vi "Kepco cfg run list.vi"(8 "error in (no error)":errorcluster {"code" format="%.0x"}, 9 "Simulation":T1, 10 "Channel parsed command info":T2, 11 "input cluster":refnum<class "KepcoBOP.lvclass">) -> (0 "error out":errorcluster, 2 "new commands":string, 3 "output cluster":refnum<class "KepcoBOP.lvclass">)   [LabVIEW 2020, in "KepcoBOP.lvclass"]
uses:
  KepcoBOP.lvclass
  channel parsed cmd cluster.ctl
  OnOffTypeDef.ctl
  KepcoBOP.lvclass/KepcoBOP.ctl
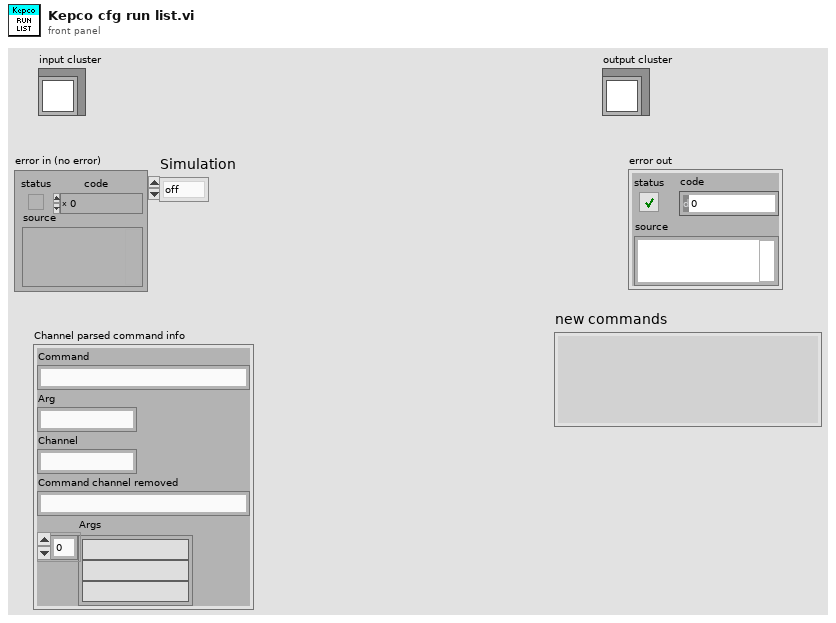
[diagram p1: front panel]
types:
  T1 = typedef "OnOffTypeDef.ctl" = enum16{"off", "on"}
  T2 = typedef "channel parsed cmd cluster.ctl" = cluster{"Command":string, "Arg":string, "Channel":string, "Command channel removed":string, "Args":string[]}
  T3 = enum16{"Fixed", "List", "Transient", "External", "Gain", "Protect"}
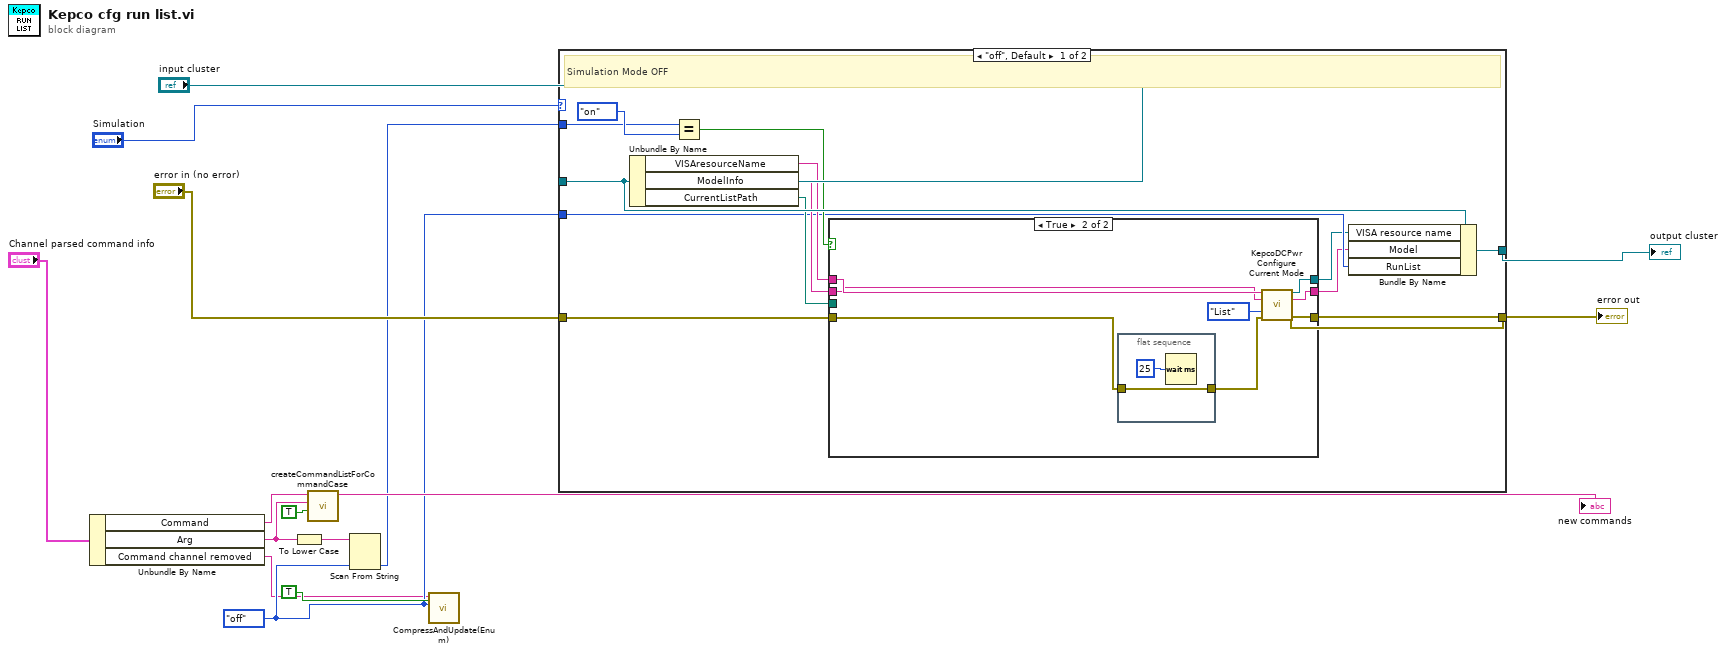
[diagram p0: block diagram]
diagram:
  w2 = enum16{"off", "on"}."off"
  n1 = Unbundle By Name("Channel parsed command info") -> ("Command"=w14:string, "Arg"=w4:string, "Command channel removed"=w1:string)
  n2 = To Lower Case(string=w4) -> (all lower case string=w5:string)
  n3 = call "createCommandListForCommandCase.vi"("immediate Check (only once)"=TRUE, "setvalue"=w4, "command"=w14) -> ("new commands"=→"new commands":string)  [unwired: 8 in]
  n4 = Scan From String(input string=w5, default 1=w2) -> (output 1=w3:enum16{"off", "on"})  [unwired: 3 in, 3 out]
  n5 = call "CompressAndUpdate(Enum).vi"("force CVT update (false)"=TRUE ("force CVT update"), "enum variant"=w2, "command or variable name"=w1) -> ()  [unwired: 8 in, 1 out]
  n6 = case shown="\"off\", Default" "Simulation" {
    tunnel: [w22 w42] -> w9
    tunnel: "input cluster" -> [w28 w43]
    tunnel: "error in (no error)" -> [w23 w42]
    tunnel: [w27 w43] -> w10
    tunnel: w3 -> [w25 _]
    tunnel: w2 -> [w18 _]
    frame "off", Default {
      # "Simulation Mode OFF"
      n7 = Unbundle By Name(w28) -> ("VISAresourceName"=w21:string, "ModelInfo"=w20:string, "CurrentListPath"=w19:path)
      n8 = Equal?(x=w25, y=enum16{"off", "on"}."on") -> (x = y?=w24:bool)
      n9 = case shown="True" w24 {
        tunnel: w23 -> [w30 w32]
        tunnel: w21 -> [w29 w34]
        tunnel: w20 -> [w31 w33]
        tunnel: [w31 w36] -> w16
        tunnel: [w30 w35] -> w22
        tunnel: w19 -> [_ _]
        tunnel: [w29 w37] -> w17
        frame False {
        }
        frame True {
          n10 = flat-sequence {
            tunnel: [w40] -> w38
            tunnel: w32 -> [w40]
            frame #0 {
              n11 = Wait (ms)(milliseconds to wait=u32 25) -> ()  [unwired: 1 out]
            }
          }
          n12 = call "KepcoDCPwr Configure Current Mode.vi"("VISA Session"=w34, "Model In"=w33, "Mode (Fixed)"=T3."List", "error in (no error)"=w38) -> ("VISA Session Out"=w37:refnum<visa-resource-name>, "Model Out"=w36:string, "error out"=w35:errorcluster)  [unwired: 8 in, 1 out]
        }
      }
      n13 = Bundle By Name(cluster=w28, "VISA resource name"=w17, "Model"=w16, "RunList"=w18) -> (w27:refnum<class "KepcoBOP.lvclass">)
    }
    frame "on" {
      # "Simulation Mode ON"
    }
  }
  "output cluster" <- w10
  "error out" <- w9
